vi "PQselect.vi"(0 "conn":u32, 1 "table":string, 2 "columns":string[](array[string]), 3 "optional clause":string, 5 "error in (no error)":errorcluster) -> (7 "PQresultStatus":T1(ring), 9 "PQresultErrorMessage":string, 11 "RowsCount":u32, 13 "ColsCount":u32, 14 "conn_out":u32, 16 "Data":string[][](array[string]), 17 "ColumnNames":string[](array[string]), 19 "error out":errorcluster)   [LabVIEW 2019, in "libpqutility.lvlib"]
doc: "SELECT columns FROM table optional clause\nResult is:\nThe Requested Data\nColumn names of Requested Data\nNumber of Rows\nNumber of Columns\n\nSee PostgreSQL c-lib dokumentation for further information.\n\nconn is the reference to the PostgreSQL connection"
uses:
  libpqutility.lvlib
  libpqlv/src/PQnfields.vi
  libpqlv/src/PQntuples.vi
  libpqlv/src/PQgetvalue.vi
  libpqlv/src/PQfname.vi
  libpqlv/libpqlv.lvlib
panel:
  out "selectstring":string
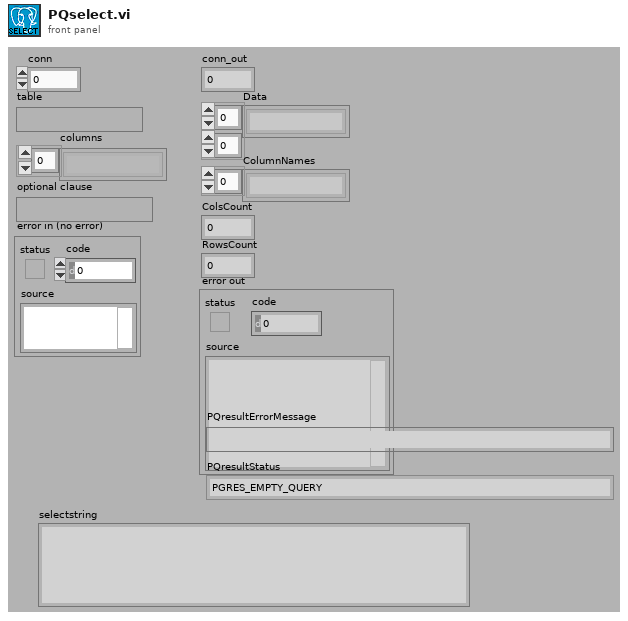
[diagram p1: front panel]
types:
  T1 = enum16{"PGRES_EMPTY_QUERY", "PGRES_COMMAND_OK", "PGRES_TUPLES_OK", "PGRES_COPY_OUT", "PGRES_COPY_IN", "PGRES_BAD_RESPONSE", "PGRES_NONFATAL_ERROR", "PGRES_FATAL_ERROR"}
  T2 = enum32{"PGRES_EMPTY_QUERY", "PGRES_COMMAND_OK", "PGRES_TUPLES_OK", "PGRES_COPY_OUT", "PGRES_COPY_IN", "PGRES_BAD_RESPONSE", "PGRES_NONFATAL_ERROR", "PGRES_FATAL_ERROR"}
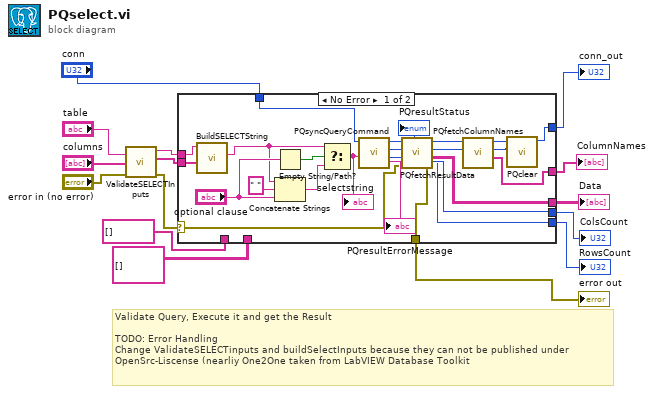
[diagram p0: block diagram]
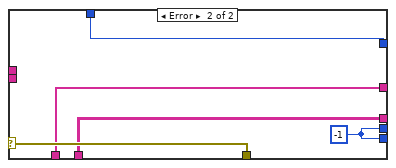
[diagram p2: hidden frame]
diagram:
  # "Validate Query, Execute it and get the Result\n\nTODO: Error Handling\nChange ValidateSELECTinputs and buildSelectInputs because they can not be published under \nOpenSrc-Liscense (nearliy One2One taken from LabVIEW Database Toolkit"
  n1 = call "ValidateSELECTInputs.vi"("error in (no error)"="error in (no error)", "columns"="columns", "table"="table") -> ("error out"=w8:errorcluster, "columns out"=w9:string[], "table out"=w10:string)  [unwired: 6 in]
  n2 = case shown="No Error" w8 {
    selector: w8 -> [w17 w44]
    tunnel: w9 -> [w31 _]
    tunnel: w10 -> [w30 _]
    tunnel: [w16 w44] -> w1
    tunnel: "conn" -> [w35 w42]
    tunnel: [w27 w43] -> w15
    tunnel: string[][] [] ("null") -> [_ w43]
    tunnel: [w28 w42] -> w6
    tunnel: [w22 w41] -> w5
    tunnel: string[] [] ("ColumnNames") -> [_ w41]
    tunnel: [w21 w40] -> w3
    tunnel: [w20 w40] -> w2
    frame No Error {
      n3 = call "BuildSELECTString.vi"("columns"=w31, "table"=w30) -> ("select query"=w32:string)  [unwired: 9 in]
      n4 = Empty String/Path?(string/path="optional clause") -> (empty?=w39:bool)
      n5 = Concatenate Strings(w32, " " ("Substring"), "optional clause") -> (w38:string)
      n6 = Select(t=w32, s=w39, f=w38) -> (s? t:f=w34:string)
      "selectstring" <- w34
      n7 = call "PQsyncQueryCommand.vi"("query"=w34, "conn"=w35) -> ("PQresultStatus"=→"PQresultStatus":T2, "PGresult"=w33:u32, "conn out"=w29:u32, "PQresultErrorMessage"=→"PQresultErrorMessage":string)  [unwired: 5 in, 1 out]
      n8 = call "PQfetchResultData.vi"("error in"=w17, "res"=w33, "conn"=w29) -> ("error out"=w16:errorcluster, "Data"=w27:string[][], "res_out"=w26:u32, "conn_out"=w25:u32, "PQnFields"=w20:i32, "PQnTuples"=w21:i32)  [unwired: 3 in]
      n9 = call "PQfetchColumnNames.vi"("res"=w26, "conn"=w25) -> ("ColumnNames"=w22:string[], "res_out"=w23:u32, "conn_out"=w24:u32)  [unwired: 4 in, 1 out]
      n10 = call "PQclear.vi"("res"=w23, "conn"=w24) -> ("conn_out"=w28:u32)  [unwired: 8 in, 1 out]
    }
    frame Error {
      w40 = -1 ("PQnFields")
    }
  }
  "error out" <- w1
  "Data" <- w15
  "conn_out" <- w6
  "ColumnNames" <- w5
  "ColsCount" <- w3
  "RowsCount" <- w2
